vi "Timer Mode Configuration.vi"(8 "error in":errorcluster, 9 "TimerValues":dbl[](array[numeric]) format="%.2f", 10 "TimerModes":string[](array[string]), 11 "Handle In":i32) -> (0 "error out":errorcluster, 3 "Handle Out":i32)   [LabVIEW 2021]
panel:
  # "Timer Mode Strings:\nLJ_tmPWM16\nLJ_tmPWM8\nLJ_tmRISINGEDGES32\nLJ_tmFALLINGEDGES32\nLJ_tmDUTYCYCLE\nLJ_tmFIRMCOUNTER\nLJ_tmFIRMCOUNTERDEBOUNCE\nLJ_tmFREQOUT\nLJ_tmQUAD\nLJ_tmTIMERSTOP\nLJ_tmSYSTIMERLOW\nLJ_tmSYSTIMERHIGH\nLJ_tmRISINGEDGES16\nLJ_tmFALLINGEDGES16"
  # "Timer0\n\nTimer1\n\nTimer2\n\nTimer3\n\nTimer4\n\nTimer5"
  # "The number of timers to configure is\ndetermined by the number of elements\nin the TimerModes array."
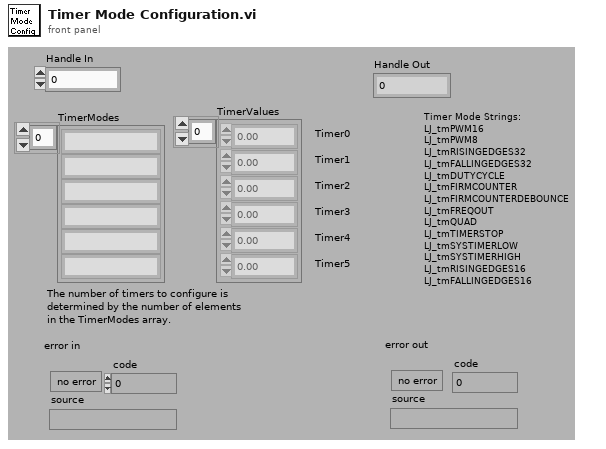
[diagram p1: front panel]
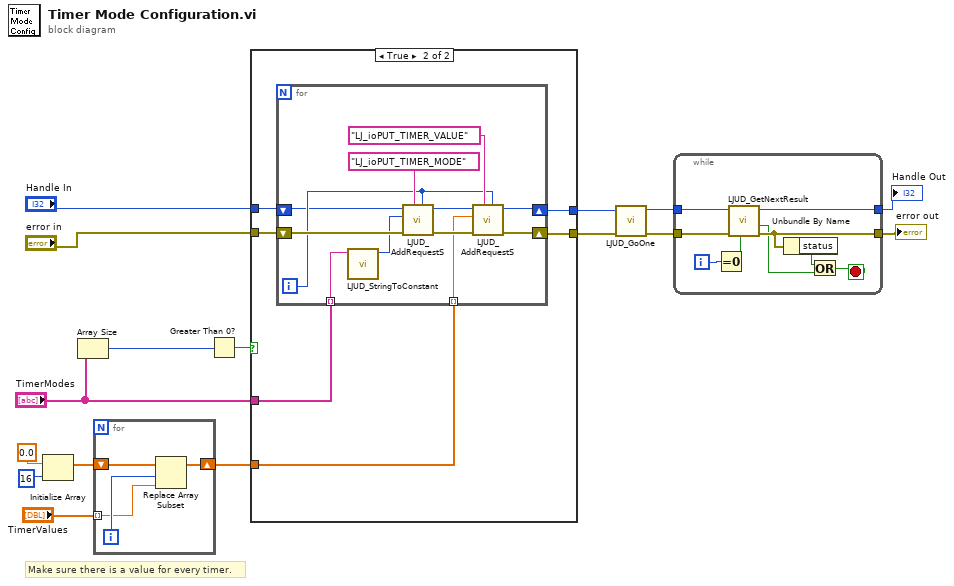
[diagram p0: block diagram]
diagram:
  # "Make sure there is a value for every timer."
  n1 = Initialize Array(0.0, 16 ("Element Data")) -> (w5:dbl[])
  n2 = Array Size(array="TimerModes") -> (size(s)=w6:i32)
  n3 = for {
    shift-right: [w20] -> w1
    shift-left: w5 -> [w19]
    tunnel: "TimerValues" -> [w17] mode=indexing
    i -> [w18]
    n4 = Replace Array Subset(array=w19, new element=w17, index=w18) -> (w20:dbl[])
  }
  n5 = Greater Than 0?(x=w6) -> (x > 0?=w7:bool)
  n6 = case shown="True" w7 {
    tunnel: "error in" -> [w22 w28]
    tunnel: "TimerModes" -> [_ w27]
    tunnel: w1 -> [_ w26]
    tunnel: [w22 w25] -> w8
    tunnel: "Handle In" -> [w21 w24]
    tunnel: [w21 w23] -> w9
    frame False {
    }
    frame True {
      n7 = for {
        shift-right: [w33] -> w25
        shift-left: w28 -> [w36]
        tunnel: w27 -> [w30] mode=indexing
        tunnel: w26 -> [w35] mode=indexing
        shift-right: [w31] -> w23
        shift-left: w24 -> [w32]
        i -> [w34]
        n8 = call "LJUD_StringToConstant.vi"("String"=w30) -> ("Constant Number"=w29:i32)  [unwired: 9 in, 1 out]
        n9 = call "LJUD_AddRequestS.vi"("Channel"=w34, "IOType"="LJ_ioPUT_TIMER_MODE", "error in"=w36, "Value"=w29, "Handle In"=w32) -> ("error out"=w38:errorcluster, "Handle Out"=w37:i32)  [unwired: 5 in]
        n10 = call "LJUD_AddRequestS.vi"("Channel"=w34, "IOType"="LJ_ioPUT_TIMER_VALUE", "error in"=w38, "Value"=w35, "Handle In"=w37) -> ("error out"=w33:errorcluster, "Handle Out"=w31:i32)  [unwired: 5 in]
      }
    }
  }
  n11 = call "LJUD_GoOne.vi"("error in"=w8, "Handle In"=w9) -> ("error out"=w15:errorcluster, "Handle Out"=w16:i32)  [unwired: 8 in]
  n12 = while {
    tunnel: [w43] -> w13
    tunnel: [w45] -> w14
    tunnel: w16 -> [w46]
    tunnel: w15 -> [w47]
    i -> [w42]
    stop <- w49 stop-if-true
    n13 = Equal To 0?(x=w42) -> (x = 0?=w48:bool)
    n14 = call "LJUD_GetNextResult.vi"("GetFirst"=w48, "error in"=w47, "Handle In"=w46) -> ("error out"=w45:errorcluster, "LJE_NO_MORE_DATA_AVAILABLE"=w41:bool, "Handle Out"=w43:i32)  [unwired: 3 in, 3 out]
    n15 = Unbundle By Name(w45) -> ("status"=w44:bool)
    n16 = Or(x=w44, y=w41) -> (x .or. y?=w49:bool)
  }
  "error out" <- w14
  "Handle Out" <- w13
